vi "execute_initial_value_policy.vi"(8 "error in (no error)":errorcluster, 9 "Last Publish Time":timestamp, 10 "Last Topic Value":variant, 11 "WriteWhenVisibleSubscription In":refnum<class "WriteWhenVisibleSubscription.lvclass">) -> (0 "error out":errorcluster, 3 "WriteWhenVisibleSubscription Out":refnum<class "WriteWhenVisibleSubscription.lvclass">)   [LabVIEW 2017, in "SubscriptionPolicy.lvlib" / "WriteWhenVisibleSubscription.lvclass"]
uses:
  WriteWhenVisibleSubscription.lvclass
  C:/Git/mva-framework/Framework/IMediator/ISubscriptionPolicy/ISubscriptionPolicy.lvclass
  WriteWhenVisibleSubscription.lvclass/WriteWhenVisibleSubscription.ctl
  IMediator/ISubscriptionPolicy/ISubscriptionPolicy.lvclass/ISubscriptionPolicy.ctl
  IMediator/ITransport/ITransport.lvclass
  IMediator/ISubscriptionPolicy/ISubscriptionPolicy.lvclass
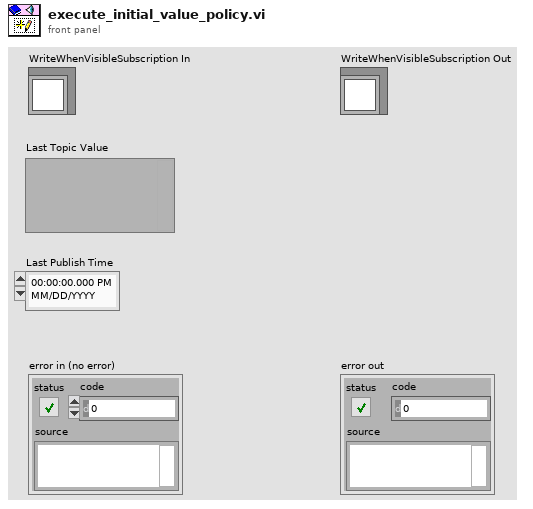
[diagram p1: front panel]
types:
  T1 = enum32{"Invalid", "Standard", "Closed", "Hidden", "Minimized", "Maximized"}
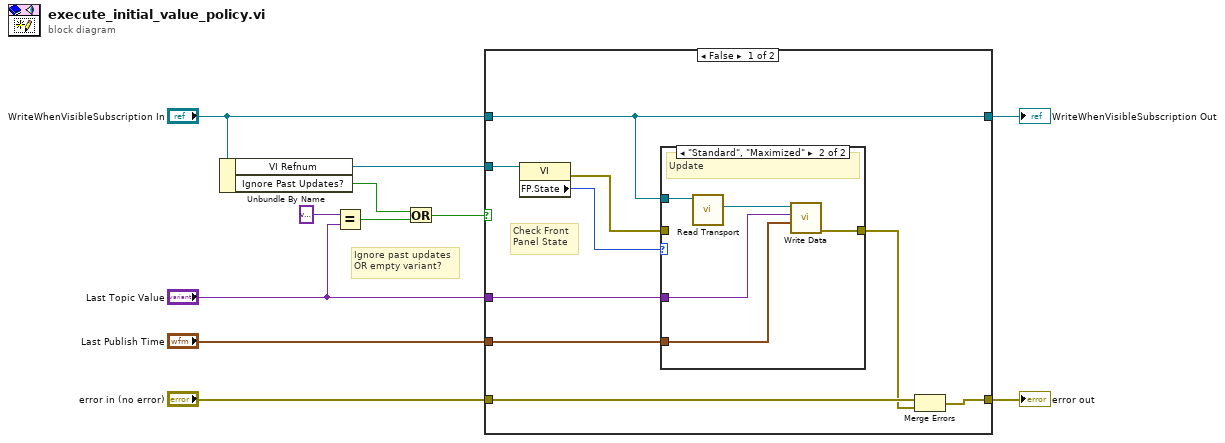
[diagram p0: block diagram]
diagram:
  # "Ignore past updates\nOR empty variant?"
  n1 = Unbundle By Name("WriteWhenVisibleSubscription In") -> ("VI Refnum"=w1:refnum<vi>, "Ignore Past Updates?"=w4:bool)
  n2 = Equal?(x=variant, y="Last Topic Value") -> (x = y?=w5:bool)
  n3 = Or(x=w4, y=w5) -> (x .or. y?=w3:bool)
  n4 = case shown="False" w3 {
    tunnel: "error in (no error)" -> [w20 w27]
    tunnel: "Last Topic Value" -> [w19 _]
    tunnel: "Last Publish Time" -> [w18 _]
    tunnel: [w17 w27] -> w9
    tunnel: "WriteWhenVisibleSubscription In" -> [w15 w28]
    tunnel: [w15 w28] -> w8
    tunnel: w1 -> [w14 _]
    frame False {
      # "Check Front\nPanel State"
      n5 = property class="VI"(reference=w14) -> (error out=w12:errorcluster, "FP.State"=w13:T1)  [unwired: 1 in, 1 out]
      n6 = case shown="\"Standard\", \"Maximized\"" w13 {
        tunnel: w19 -> [_ w26]
        tunnel: w18 -> [_ w25]
        tunnel: [w21 w24] -> w16
        tunnel: w15 -> [_ w22]
        tunnel: w12 -> [w21 _]
        frame Default {
          # "No update"
        }
        frame "Standard", "Maximized" {
          # "Update"
          n7 = call "Read Transport.vi"("ISubscriptionPolicy in"=w22) -> ("Transport"=w23:refnum<class "ITransport.lvclass">)  [unwired: 10 in]
          n8 = call-dynamic "Write Data.vi"("Publication Time"=w25, "Value"=w26, "ITransport in"=w23) -> ("error out"=w24:errorcluster)  [unwired: 7 in, 1 out]
        }
      }
      n9 = Merge Errors(w20, w16) -> (w17:errorcluster)
    }
    frame True {
    }
  }
  "error out" <- w9
  "WriteWhenVisibleSubscription Out" <- w8
